vi "Register Connection Event Callbacks.vi"(8 "error in (no error)":errorcluster, 11 "TwinCAT ADS in":refnum<class "TwinCAT ADS.lvclass">) -> (0 "error out":errorcluster, 3 "TwinCAT ADS out":refnum<class "TwinCAT ADS.lvclass">)   [LabVIEW 2018, in "TwinCAT ADS.lvclass"]
uses:
  TwinCAT ADS.lvclass
  TwinCAT ADS.lvclass/TwinCAT ADS.ctl
  TwinCAT.Ads
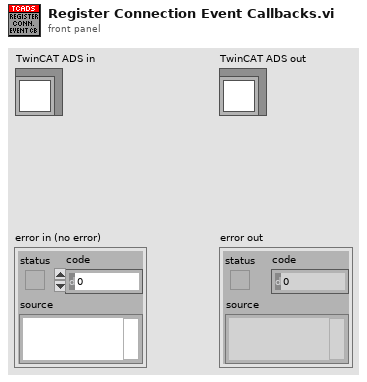
[diagram p1: front panel]
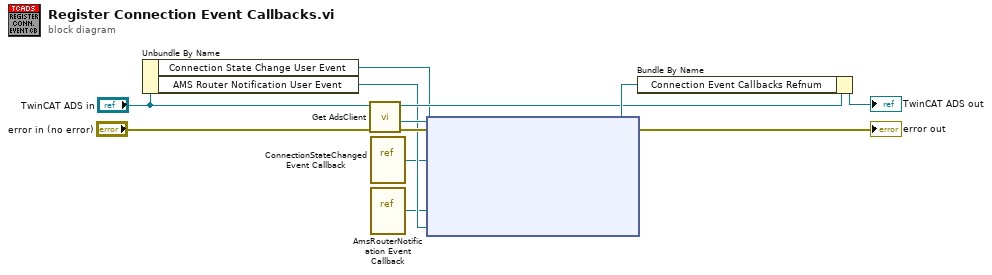
[diagram p0: block diagram]
diagram:
  n1 = Unbundle By Name("TwinCAT ADS in") -> ("Connection State Change User Event"=w4:refnum<user-event>, "AMS Router Notification User Event"=w5:refnum<user-event>)
  n2 = call "Get AdsClient.vi"("error in (no error)"="error in (no error)", "TwinCAT ADS in"="TwinCAT ADS in") -> ("error out"=w12:errorcluster, ".NET TcAdsClient"=w11:refnum<k24>, "TwinCAT ADS out"=w6:refnum<class "TwinCAT ADS.lvclass">)  [unwired: 7 in]
  n3 = vi-ref "ConnectionStateChanged Event Callback.vi"() -> ("vi reference"=w3:refnum<vi>)
  n4 = vi-ref "AmsRouterNotification Event Callback.vi"() -> ("vi reference"=w2:refnum<vi>)
  n5 = node(w12, w11, w3, w4, w11, w2, w5) -> (w8:refnum<k27>, →"error out":errorcluster)  [unwired: 1 in]
  n6 = Bundle By Name(cluster=w6, "Connection Event Callbacks Refnum"=w8) -> (→"TwinCAT ADS out":refnum<class "TwinCAT ADS.lvclass">)
